vi "Write.vi"(8 "error in (no error)":errorcluster, 10 "Data":string, 11 "Connection in":refnum<class "Connection.lvclass">) -> (0 "error out":errorcluster, 3 "Connection out":refnum<class "Connection.lvclass">)   [LabVIEW 2022 SP3, in "TcpSocket.lvlib" / "Connection.lvclass"]
uses:
  Connection.lvclass
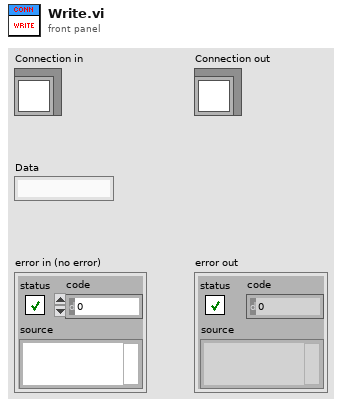
[diagram p1: front panel]
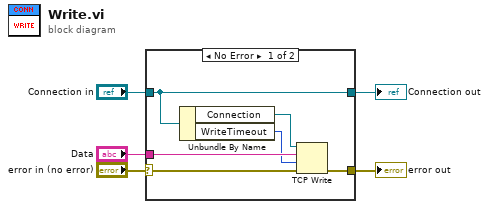
[diagram p0: block diagram]
diagram:
  n1 = case shown="No Error" "error in (no error)" {
    selector: "error in (no error)" -> [w8 w13]
    tunnel: [w7 w13] -> w4
    tunnel: [w11 w12] -> w2
    tunnel: "Connection in" -> [w11 w12]
    tunnel: "Data" -> [w9 _]
    frame No Error {
      n2 = Unbundle By Name(w11) -> ("Connection"=w10:refnum<k5>, "WriteTimeout"=w6:i32)
      n3 = TCP Write(connection ID=w10, data in=w9, error in (no error)=w8, 9:w6) -> (error out=w7:errorcluster)  [unwired: 2 out]
    }
    frame Error {
    }
  }
  "error out" <- w4
  "Connection out" <- w2
